vi "Dashboard_Main_Fixed_1280_768.vi"() -> ()   [LabVIEW 2023]
uses:
  2025ReefBot/Intake/IntakeStates.ctl
  2025ReefBot/NewAuto/NewAutoStepTypeEnum.ctl
  <vilib>/event_ctls.llb/eventvkey.ctl
  Dash_Globals.vi
  <vilib>/Rock Robotics/Network Tables/NT Read Boolean.vi
  <vilib>/Rock Robotics/Network Tables/NT Write Boolean.vi
  <vilib>/Rock Robotics/WPI/Dashboard/WPI_DashboardLogging Global.vi
  <vilib>/Rock Robotics/WPI/ThirdParty/JAS_Junk/TrajLib/Trajectory_Library.lvlib
panel:
  in  "Camera Settings Right":T1={"Frame Rate"=30, "Compression"=30, "Size"=1, "DB Camera Config"=FALSE} {"Frame Rate" scale=1.0..30.0; "Compression" scale=100.0..-1.0; "Size" items=["640x480", "320x240", "160x120"]}
  in  "Camera Name Right":string(combo)="No Camera Selection"
  out "Camera Perf":string
  in  "Camera Settings":T1={"Frame Rate"=30, "Compression"=30, "Size"=1, "DB Camera Config"=FALSE} {"Frame Rate" scale=1.0..30.0; "Compression" scale=100.0..-1.0; "Size" items=["640x480", "320x240", "160x120"]}
  in  "TCP":refnum<k5>
  in  "Rec Mode":enum32{"Stop", "Record", "Playback"}(radio)
  out "Robot IP":string
  out "Image Message":string="Timeout in Camera Communications"
  in  "Dashboard Tab":T2(tab)
  out "Human Fast Turn":bool
  out "H Traj Orient Deg":dbl format="%11.2f"
  out "H Traj Y Ft":dbl format="%11.2f"
  out "H Traj X Ft":dbl format="%11.2f"
  out "Human Slow Mode":bool
  out "Human Field Orient":bool
  out "A String":string
  out "P3":dbl format="%11.2f"
  out "Function":T3
  out "A Step":i64 format="%11.0f"
  out "P2":dbl format="%11.2f"
  out "P1":dbl format="%11.2f"
  out "TO":dbl format="%11.2f"
  out "Vision Targets Found":bool
  out "Climb Position":dbl format="%15.2f"
  out "Climb Status":string
  out "Fully Pulled":bool
  out "Fully Reached":bool
  out "Intake State":T4
  out "Have Algae":bool
  out "Have Coral":bool
  out "W PV":dbl(slide) scale=-90.0..90.0
  out "W SP":dbl(slide) scale=-90.0..90.0
  out "W Hi Clamp":bool
  out "W Lo Clamp":bool
  out "W On Tgt":bool
  out "W Motor":dbl format="%11.2f"
  out "W Pos Deg":dbl format="%12.1f"
  out "W Dmd Deg":dbl format="%12.1f"
  out "I PV":dbl(slide) scale=0.0..26.0
  out "I SP":dbl(slide) scale=0.0..26.0
  out "I Lo Clamp":bool
  out "I Lo Lim":bool
  out "I Hi Lim":bool
  out "I On Tgt":bool
  out "I Motor":dbl format="%11.2f"
  out "I Pos In":dbl format="%12.1f"
  out "I Dmd In":dbl format="%12.1f"
  in  "Select Auto":string(combo)="Select Autonomous ..."
  out "NT Connection":bool
  out "Mode":T5(ring)=enum."Auto Disabled"
  out "Right Camera Perf":cluster{"Bandwidth (Mbps)":dbl, "FPS":dbl}
  out "Selected Auto":string
  out "O PV":dbl(slide) scale=0.0..52.0
  out "O SP":dbl(slide) scale=0.0..52.0
  out "O Lo Lim":bool
  out "O Hi Lim":bool
  out "O On Tgt":bool
  out "O Motor":dbl format="%11.2f"
  out "O Pos In":dbl format="%12.1f"
  out "O Dmd In":dbl format="%12.1f"
  out "Camera Image Right":T6(plugin-control)
  out "AlgaeIntakeFB":dbl
  out "AlgaeHoldFB":dbl
  in  "AlgaeIntake":dbl
  in  "AlgaeHold":dbl
  in  "AlgaeTune":bool
  out "Max Amb FB":dbl
  in  "Max Amb":dbl
  out "I Orient Deg FB":dbl
  in  "Init Orient Deg":dbl
  out "InitYPosFt FB":dbl
  in  "InitYPos Ft":dbl
  in  "Vision Update":bool
  out "InitXPos Ft FB":dbl
  in  "InitXPos Ft":dbl
  out "RL Enable FB":bool
  in  "RL Enable":bool
  out "Y Acc M/S2 FB":dbl
  in  "Y Acc M/S2":dbl
  in  "RL Update":bool
  out "X Acc M/S2 FB":dbl
  in  "X Acc M/S2":dbl
  in  "RA Update":bool
  out "R Starting Angle FB":dbl
  in  "R Starting Angle":dbl
  in  "LQR":bool
  in  "Filter":bool
  out "Wrist Chart":T7(graph)
  out "Kp Calc":dbl
  out "Kg FB":dbl
  in  "Kg":dbl
  out "Kd FB":dbl format="%#_7g"
  in  "Kd":dbl format="%#_7g"
  out "Output Max FB":dbl
  in  "Output Max":dbl
  out "Output DB FB":dbl
  in  "Output DB":dbl
  out "Error DB FB":dbl
  in  "Error DB":dbl
  in  "WR Tune Update":bool
  out "Error Thres FB":dbl
  in  "Error Thres":dbl
  out "Filt FB":bool
  out "LQR FB":bool
  in  "Test Slider":dbl(slide) scale=0.0..100.0 scale format="%#_3g"
  in  "On/Off":bool caption="Solenoid"
  in  "Test Name":u16(ring) items=["Select the test to run..."]
  in  "Test Tree":string(tree)
  in  "Motor":cluster{"Value":dbl, "Enable":bool} {"Value" scale=-1.0..1.0 scale format="%#_3g"}
  out "Progress":T8 {"Test Progress" scale=0.0..100.0}
  in  "Rev/Fwd":cluster{"Forward":bool, "Reverse":bool}
  in  "Test Ring":u16(ring) items=["Monochrome", "Color"]
  in  "CheckList":i32(listbox)
  out "Tree":string(tree)
  out "Camera Image":T6(plugin-control)
  out "Background":bool
  in  "Camera Name":string(combo)="No Camera Selection"
  # "HW"
  # "HW"
  # "Human"
  # "Auto"
  # "VISION"
  # "CLIMB"
  # "INTAKE"
  # "WRIST"
  # "INNER ELEV"
  # "OUTER ELEV"
  # "Vision Tuning"
  # "Drive Rate Limiting"
  # "Initial Robot Angle"
  # "Wrist Tuning"
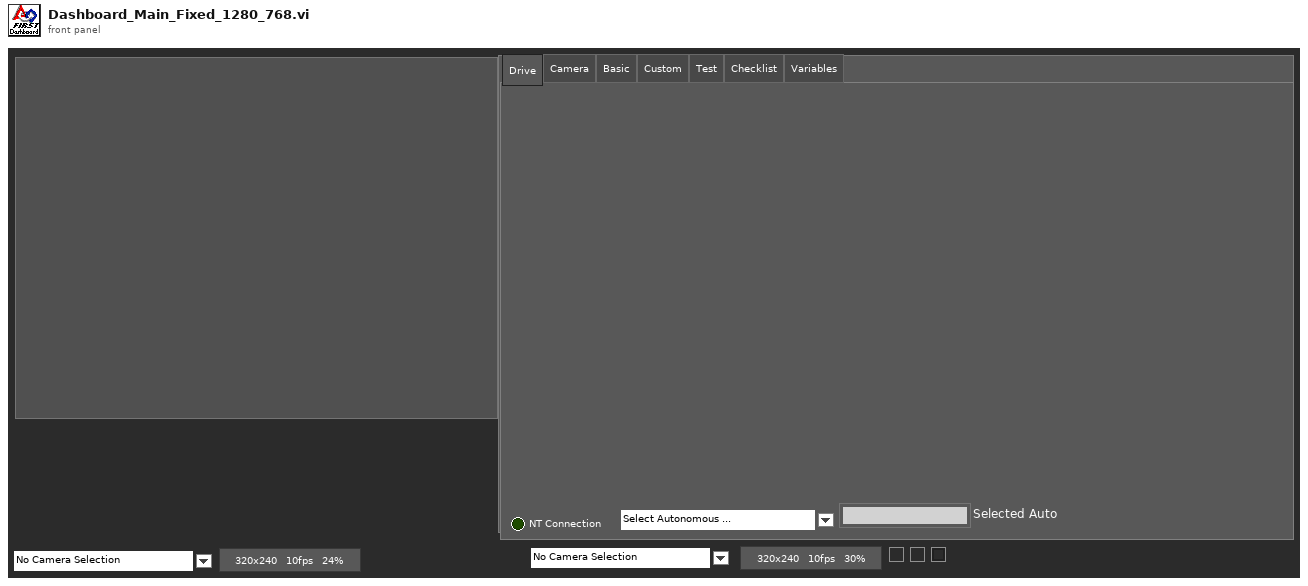
[diagram p1: front panel]
types:
  T1 = cluster{"Frame Rate":i32, "Compression":i32, "Size":u16, "DB Camera Config":bool}
  T2 = enum32{"Drive", "Camera", "Basic", "Custom", "Test", "Checklist", "Variables"}
  T3 = typedef "NewAutoStepTypeEnum.ctl" = enum16{"DriveStraight", "DriveTurn", "FollowAbsoluteTrajectory", "FollowRelativeTrajectory", "AutoWait", "ElevToRest", "ElevToFloor", "ElevToSource", "ElevToL1", "ElevToL2", "ElevToL3", "ElevToL4", "ElevToAlgae1", "ElevToAlgae2", "ElevToBarge", "ElevCancel", "IntakeCoral", "IntakeAlgae", "IntakeDepositCoral", "IntakeDepositAlgae", "IntakeCancel", "ElevRestWait", "ElevFloorWait", "ElevSourceWait", "ElevL1Wait", "ElevL2Wait", "ElevAlgae1Wait", "ElevL3Wait", "ElevAlgae2Wait", "ElevL4Wait", "ElevBargeWait", "IntakeWait", "FollowAbsTrajWithTimedCmd", "FollowRelTrajWithTimedCmd"}
  T4 = typedef "IntakeStates.ctl" = enum16{"Start", "WaitForCommand", "IntakeCoral", "IntakeAlgae", "WaitForCoral", "WaitForAlgae", "DepositCoral", "DepositAlgae", "DepositCoralTimer", "DepositAlgaeTimer"}
  T5 = enum8{"Tele-Op Disabled", "Tele-Op Enabled", "Auto Disabled", "Auto Enabled", "Test Disabled", "Test Enabled", "Disconnected", "No Code", "E-Stop"}
  T6 = typedef "IMAQ Image.ctl" = refnum<image>
  T7 = cluster{"WristSetpointDeg":dbl, "WristPosDeg":dbl, "WristMotorDmd":dbl, "WristGravityCompMotorDmd":dbl}
  T8 = cluster{"Test Progress":u8, "Test Progress Text":string}
  T9 = cluster{"Save Path":path, "Interval (s)":dbl, "Keep":i32}
  T10 = typedef "Image Type" = u32
  T11 = enum32{"Drive", "Camera", "Basic", "Custom", "Test", "Commands", "Checklist", "Variables"}
  T12 = cluster{"Error Strings":string, "Disable Counts":cluster{u16, u16}, "Rail Faults":cluster{u16, u16, u16}, "Robot IP":string, "DB Mode":u8, "Event Info":cluster{"Name":string, "Type":u8, "Number":u16, "Replay":u8}}
  T13 = cluster{"Storage":cluster{"Disk Free":u64, "RAM Block":u32, "RAM free":u32}, "CPU Utilization":cluster{"CPU % ISR":sgl, "CPU % Time Crit":sgl, "CPU % Timed Str":sgl, "CPU % High":sgl, "CPU % Above":sgl, "CPU % Normal":sgl, "CPU % Low":sgl}, "CAN":cluster{"% Bus Utilization":sgl, "Bus Off Cnt":u32, "TX_FIFO Full Cnt":u32, "Receive Error Cnt":u8, "Transmit Error Cnt":u8}, "HID":cluster{"HID Outputs":u32, "Rumble Low":u16, "Rumble High":u16}[]}
  T14 = cluster{"Status bits":cluster{"Test Mode":bool, "Autonomous":bool, "Enabled":bool, "Code Start":bool, "Brownout":bool, "Reserved 2":bool, "Reserved 3":bool, "E-Stop":bool}, "Code Trace":cluster{"Disabled":bool, "TeleOp":bool, "Auto":bool, "Test":bool}, "Controller Type":enum16{"unknown", "cRIO", "roboRio"}, "Code?":enum16{"unknown", "noCode", "code"}, "Battery V":dbl}
  T15 = cluster{"Control Bits":cluster{"TestMode":bool, "Autonomous":bool, "Enabled":bool, "FMS Present":bool, bool, bool, bool, "E-Stop":bool}, "Team Station ":u8, "Countdown":sgl, "Joystick Values":cluster{"Axes":dbl[], "Buttons":bool[], "POVs":i16[]}[]}
  T16 = cluster{"Camera Image":refnum<vi>, "Dashboard Tab":refnum<vi>, "Background":refnum<vi>, "Rec Mode":refnum<vi>, "Test Slider":refnum<vi>, "On/Off ":refnum<vi>, "Test Ring":refnum<vi>, "Rev/Fwd":refnum<vi>, "Test Name":refnum<vi>, "Motor":refnum<vi>, "Progress":refnum<vi>, "CheckList":refnum<vi>, "Tree":refnum<vi>, "Test Tree":refnum<vi>, "Camera Settings":refnum<vi>, "Camera Name":refnum<vi>, "Camera Perf":refnum<vi>, "Camera Settings Right":refnum<vi>, "Camera Name Right":refnum<vi>, "Camera Image Right":refnum<vi>}
  T17 = cluster{"Global Rectangle":i32[], "Contours":cluster{"Contour Type":u32, "ROI Type":u32, "Points":i32[]}[]}
  T18 = cluster{"Camera Name":string, string, "Saved DB Images Info":cluster{"Save Path":path, "Interval (s)":dbl, "Keep":i32}}
  T19 = cluster{"Camera Name Right":string, string, "Saved DB Images Info":cluster{"Save Path":path, "Interval (s)":dbl, "Keep":i32}}
  T20 = cluster{"Operation":enum16{"Update", "Clear"}, "Color Box":u32}[]
  T21 = typedef "eventvkey.ctl" = enum16{"ASCII", "Enter", "Return", "Shift", "Ctrl", "Alt", "Cmd", "Opt", "Caps", "NumLock", "Clear", "Break", "Up", "Down", "Left", "Right", "Insert", "Delete", "Home", "End", "PageUp", "PageDown", "Escape", "Help", "Pause", "ScrollLock", "F1", "F2", "F3", "F4", "F5", "F6", "F7", "F8", "F9", "F10", "F11", "F12", "F13", "F14", "F15", "F16", "F17", "F18", "F19", "F20", "F21", "F22", "F23", "F24", "Play", "VolumeUp", "VolumeDown", "Mute", "Two Byte Char"}
  T22 = cluster{"Image Size":bool, "Image Type":bool, "Pixel Value":bool, "ROI Information":bool, "Zoom Factor":bool}
  T23 = cluster{"Operation":enum16{"Update", "Clear"}, "Color Box":u32}
  T24 = cluster{"Shift":bool, "Ctrl":bool, "Alt":bool, "Cmd":bool, "Opt":bool}
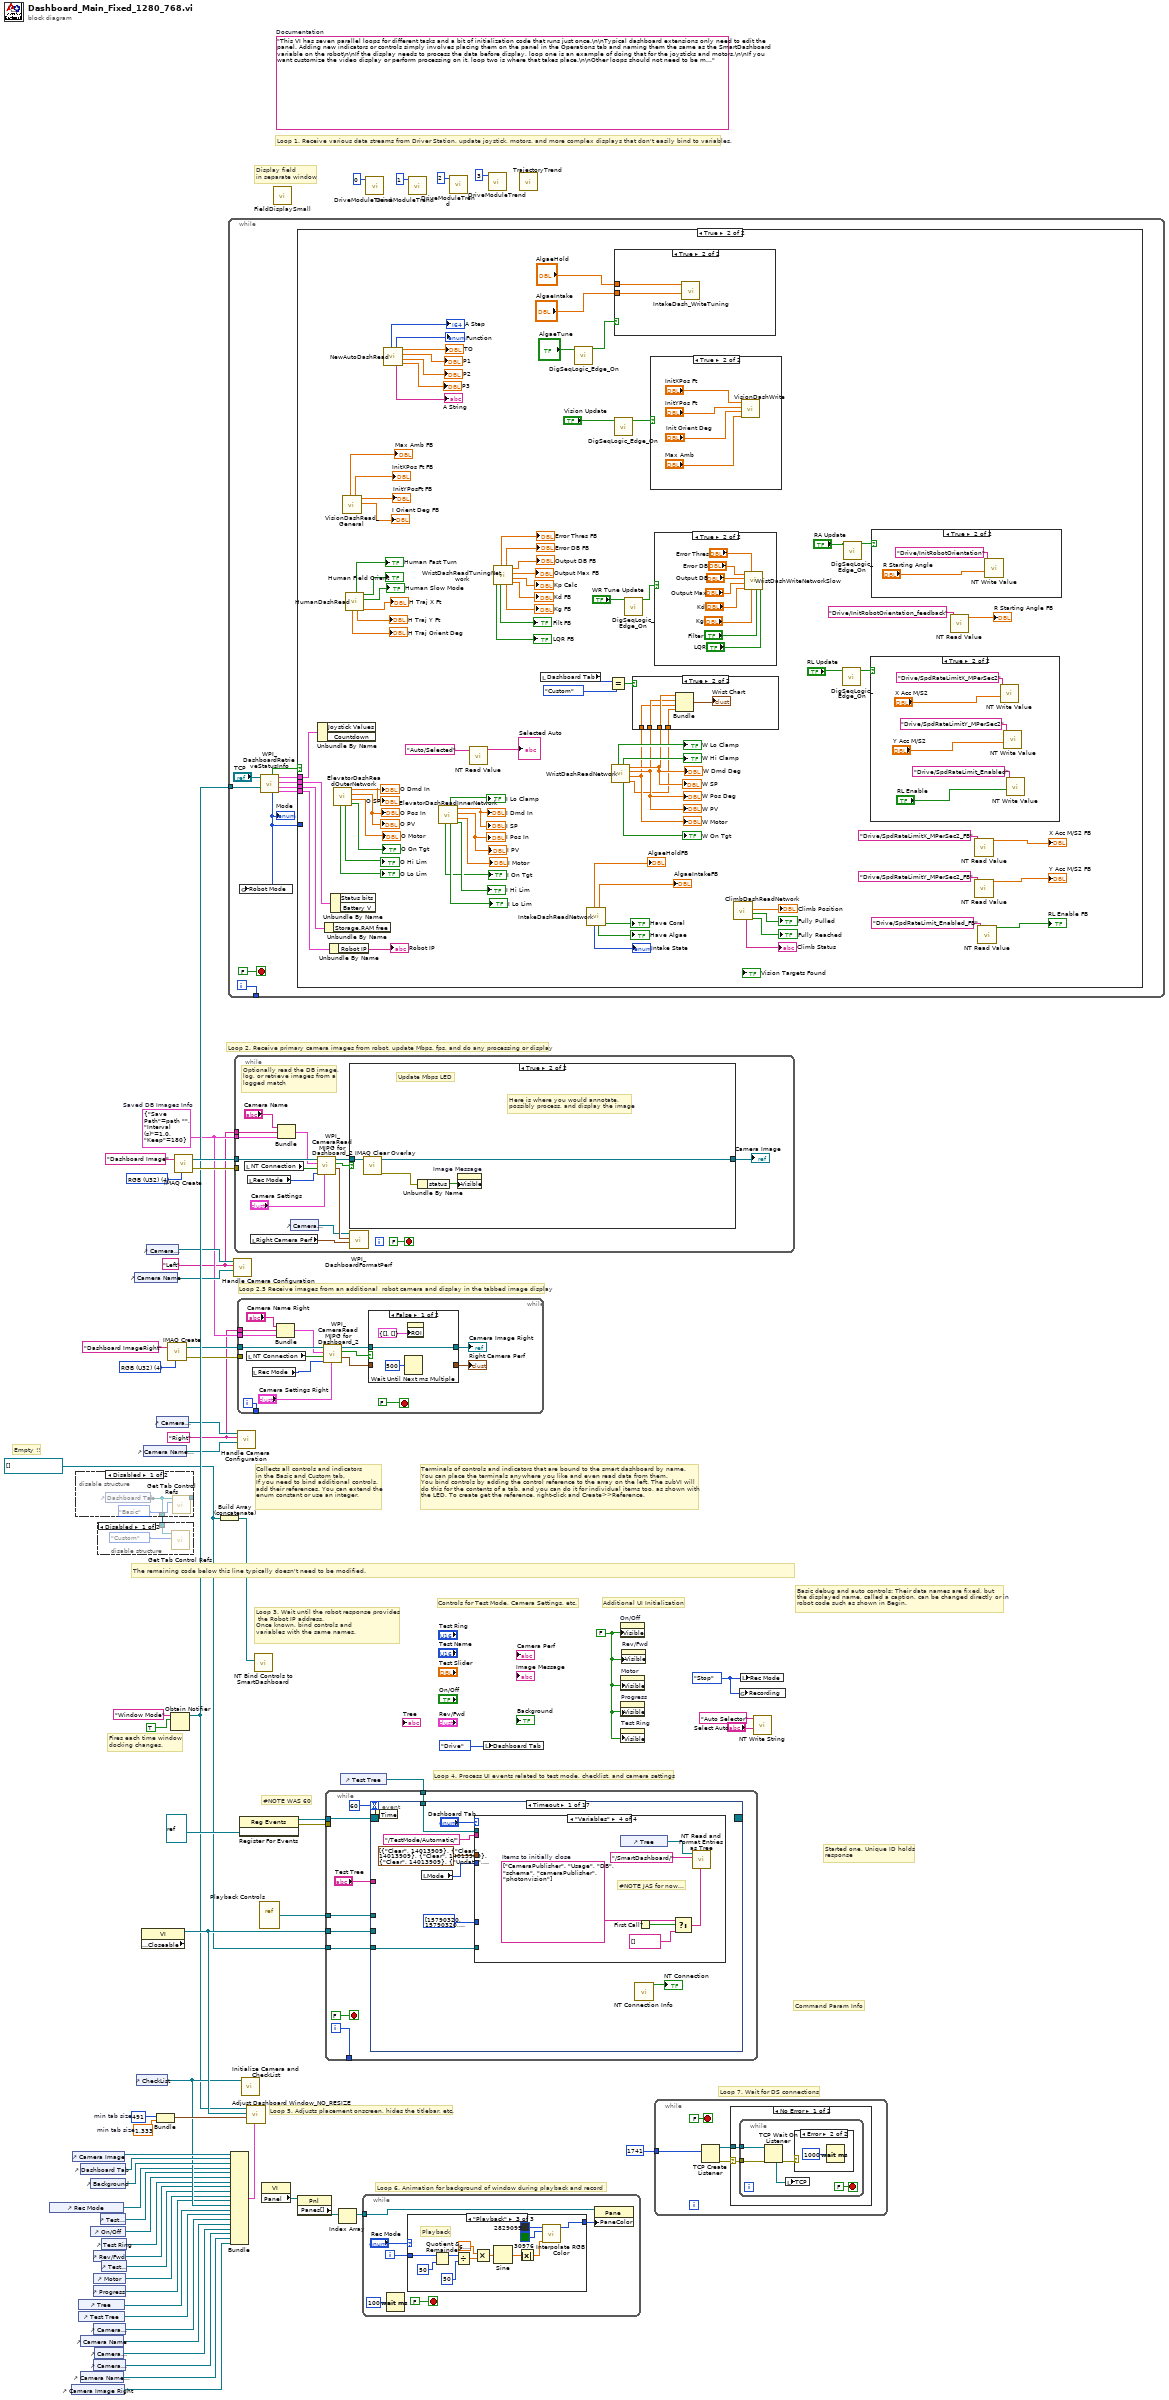
[diagram p0: block diagram]
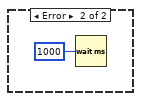
[diagram p6: hidden frame]
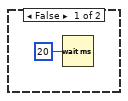
[diagram p7: hidden frame]
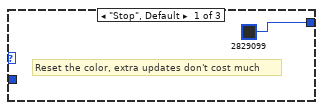
[diagram p14: hidden frame]
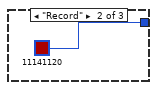
[diagram p15: hidden frame]
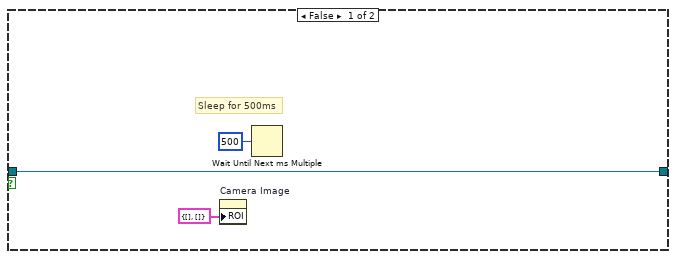
[diagram p16: hidden frame]
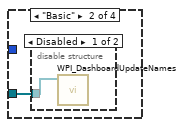
[diagram p18: hidden frame]
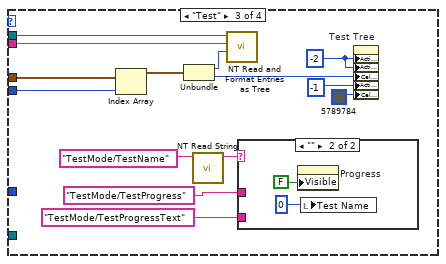
[diagram p20: hidden frame]
diagram:
  w5 = refnum<vi>[] [] ("ControlsOnPage")
  w8 = T9 {"Save Path"=path "", "Interval (s)"=1.0, "Keep"=180}  # Saved DB Images Info
  w7 = "Right"
  w6 = "Left"
  w16 = T10 4 items=["Grayscale (U8)", "Grayscale (I16)", "Grayscale (SGL)", "Complex (CSG)", "RGB (U32)", "HSL (U32)", "RGB (U64)"] ("Image Type")
  w44 = 491  # min tab size
  w43 = 1.333  # min tab size
  w50 = enum32{"Stop", "Record", "Playback"}."Stop" ("Rec Mode")
  w28 = FALSE ("Visible")
  (unwired) "This VI has seven parallel loops for different tasks and a bit of initialization code that runs just once.\n\nTypical dashboard extensions only need to edit the panel. Adding new indicators or controls simply involves placing them on the panel in the Operations tab and naming them the same as the SmartDashboard variable on the robot\n\nIf the display needs to process the data before display, loop one is an example of doing that for the joysticks and motors.\n\nIf you want customize the video display or perform processing on it, loop two is where that takes place.\n\nOther loops should not need to be modified. They are pretty standard, and document the task they perform."  # Documentation
  w64 = T10 4 items=["Grayscale (U8)", "Grayscale (I16)", "Grayscale (SGL)", "Complex (CSG)", "RGB (U32)", "HSL (U32)", "RGB (U64)"] ("Image Type")
  # "#NOTE WAS 60"
  # "Empty !!"
  # "Display field\nin separate window"
  # "Loop 2.5 Receive images from an additional  robot camera and display in the tabbed image display"
  # "Command Param Info"
  # "Started one, Unique ID holds\nresponse"
  # "Loop 7. Wait for DS connections"
  # "Basic debug and auto controls: Their data names are fixed, but\nthe displayed name, called a caption, can be changed directly or in\nrobot code such as shown in Begin."
  # "Controls for Test Mode, Camera Settings, etc."
  # "Additional UI Initialization"
  # "Loop 6. Animation for background of window during playback and record"
  # "Fires each time window\ndocking changes."
  # "Collects all controls and indicators\nin the Basic and Custom tab.\nIf you need to bind additional controls,\nadd their references. You can extend the\nenum constant or use an integer."
  # "The remaining code below this line typically doesn't need to be modified."
  # "Loop 4. Process UI events related to test mode, checklist, and camera settings"
  # "Terminals of controls and indicators that are bound to the smart dashboard by name.\nYou can place the terminals anywhere you like and even read data from them.\nYou bind controls by adding the control reference to the array on the left. The subVI will\ndo this for the contents of a tab, and you can do it for individual items too, as shown with\nthe LED. To create get the reference, right-click and Create>>Reference."
  # "Loop 3. Wait until the robot response provides\n the Robot IP address.\nOnce known, bind controls and\nvariables with the same names."
  # "Loop 5. Adjusts placement onscreen, hides the titlebar, etc."
  # "Loop 1. Receive various data streams from Driver Station, update joystick, motors, and more complex displays that don't easily bind to variables."
  # "Loop 2. Receive primary camera images from robot, update Mbps, fps, and do any processing or display"
  n1 = control-ref of="Rec Mode"() -> (w34:refnum<vi>)
  n2 = control-ref of="Camera Image Right"() -> (w9:refnum<vi>)
  n3 = control-ref of="Camera Image"() -> (w46:refnum<vi>)
  n4 = disable-structure shown="Disabled" {
    disable-tunnel: [w67 _] -> w48
    disable-tunnel: [w66 _] -> _
    frame Disabled {
      n5 = control-ref of="Dashboard Tab"() -> (w67:refnum<vi>)
      n6 = call <vilib>:"Get Tab Control Refs.vi"("Page Index"=T11."Basic" ("Dashboard Tab"), "TabControl in"=w67) -> ("ControlsOnPage"=w66:refnum<vi>[])  [unwired: 9 in]
    }
    frame Enabled {
    }
  }
  n7 = control-ref of="Tree"() -> (w38:refnum<vi>)
  n8 = control-ref of="Test Tree"() -> (w37:refnum<vi>)
  n9 = control-ref of="Dashboard Tab"() -> (w45:refnum<vi>)
  n10 = control-ref of="Camera Name"() -> (w21:refnum<vi>)
  n11 = control-ref of="Camera Name Right"() -> (w10:refnum<vi>)
  n12 = control-ref of="Background"() -> (w41:refnum<vi>)
  n13 = control-ref of="On/Off"() -> (w32:refnum<vi>)
  n14 = control-ref of="Progress"() -> (w29:refnum<vi>)
  n15 = control-ref of="Camera Settings"() -> (w22:refnum<vi>)
  n16 = control-ref of="Camera Settings Right"() -> (w11:refnum<vi>)
  n17 = control-ref of="Rev/Fwd"() -> (w30:refnum<vi>)
  n18 = control-ref of="Motor"() -> (w35:refnum<vi>)
  n19 = control-ref of="Camera Perf"() -> (w20:refnum<vi>)
  n20 = disable-structure shown="Disabled" {
    disable-tunnel: w48 -> [w69 _]
    frame Disabled {
      n21 = call <vilib>:"Get Tab Control Refs.vi"("Page Index"=T11."Custom" ("Dashboard Tab"), "TabControl in"=w69) -> ()  [unwired: 9 in, 1 out]
    }
    frame Enabled {
    }
  }
  n22 = control-ref of="Test Slider"() -> (w33:refnum<vi>)
  n23 = control-ref of="Test Ring"() -> (w31:refnum<vi>)
  n24 = control-ref of="Test Name"() -> (w36:refnum<vi>)
  n25 = control-ref of="Camera Name"() -> (w23:refnum<vi>)
  n26 = control-ref of="CheckList"() -> (w39:refnum<vi>)
  n27 = property class="VI" props=["Front Panel.Closeable"]() -> (reference out=w49:refnum<vi>)  [unwired: 2 in, 2 out]
  n28 = control-ref of="Camera Name Right"() -> (w12:refnum<vi>)
  n29 = control-ref of="Camera Settings"() -> (w24:refnum<vi>)
  n30 = control-ref of="Camera Settings Right"() -> (w13:refnum<vi>)
  n31 = Bundle("min tab size"=w44, "min tab size"=w43) -> (w42:cluster{"min tab size":i32, "min tab size":dbl})  [unwired: 1 in]
  n32 = call "IMAQ Create"("Image Name"="Dashboard ImageRight", "Image Type"=w16) -> ("New Image"=w15:T6, "error out"=w14:errorcluster)  [unwired: 2 in, 1 out]
  n33 = Obtain Notifier(name (unnamed)="Window Mode", notification data type=TRUE) -> (notifier out=w27:refnum<notifier>)  [unwired: 2 in, 2 out]
  n34 = call "IMAQ Create"("Image Name"="Dashboard Image", "Image Type"=w64) -> ("New Image"=w62:T6, "error out"=w61:errorcluster)  [unwired: 2 in, 1 out]
  n35 = Build Array (concatenate)(w5) -> (w47:refnum<vi>[])
  n36 = while {
    tunnel: [w78] -> _
    tunnel: w27 -> [w71]
    i -> [w78]
    stop <- FALSE stop-if-true
    n37 = call <vilib>:"WPI_DashboardRetrieveStatusInfo.vi"("Window Mode Notifier"=w71, "TCP Cnx"="TCP") -> ("Power and Errors"=w73:T12, "Robot Metrics"=w76:T13, "Status Info"=w77:T14, "Control Info"=w74:T15, "Robot Mode"=w70:T5, "Process?"=w75:bool)  [unwired: 4 in]
    "Mode" <- w70
    n38 = global write "Dash_Globals.vi" "Robot Mode"(w70) -> ()
    n39 = case shown="True" w75 {
      tunnel: w77 -> [_ w165]
      tunnel: w76 -> [_ w164]
      tunnel: w74 -> [_ w163]
      tunnel: w73 -> [_ w162]
      tunnel: w70 -> [_ _]
      frame False {
        n40 = Wait (ms)(milliseconds to wait=u32 20) -> ()  [unwired: 1 out]
      }
      frame True {
        n41 = Unbundle By Name(w163) -> ()  [unwired: 2 out]
        n42 = Unbundle By Name(w164) -> ()  [unwired: 1 out]
        n43 = Unbundle By Name(w162) -> ("Robot IP"=→"Robot IP":string)
        n44 = Unbundle By Name(w165) -> ()  [unwired: 2 out]
        n45 = call "ElevatorDashReadOuterNetwork.vi"() -> ("OuterOnTarget"=→"O On Tgt":bool, "OuterMotorOutput"=→"O Motor":dbl, "OuterPositionHeight"=→"O PV" →"O Pos In":dbl, "OuterPosDemandHeight"=→"O SP" →"O Dmd In":dbl, "OuterHighLimitSwitch"=→"O Hi Lim":bool, "OuterLowLimitSwitch"=→"O Lo Lim":bool)  [unwired: 6 in]
        n46 = call "VisionDashRead_General.vi"() -> ("InitOrientDeg"=→"I Orient Deg FB":dbl, "InitYFt"=→"InitYPosFt FB":dbl, "InitXFt"=→"InitXPos Ft FB":dbl, "MaxAmbiguity"=→"Max Amb FB":dbl)  [unwired: 4 in, 4 out]
        n47 = call "HumanDashRead.vi"() -> ("TrajDestX_Ft"=→"H Traj X Ft":dbl, "SlowMode"=→"Human Slow Mode":bool, "FieldOriented"=→"Human Field Orient":bool, "TrajDestY_Ft"=→"H Traj Y Ft":dbl, "FastMode"=→"Human Fast Turn":bool, "TrajDestAng_Deg"=→"H Traj Orient Deg":dbl)  [unwired: 5 in, 1 out]
        n48 = call "NewAutoDashRead.vi"() -> ("P3"=→"P3":dbl, "P2"=→"P2":dbl, "P1"=→"P1":dbl, "Timeout"=→"TO":dbl, "StepString"=→"A String":string, "StepType"=→"Function":T3, "StepIndex"=→"A Step":i64)  [unwired: 5 in]
        n49 = call "ElevatorDashReadInnerNetwork.vi"() -> ("Stage3HighLimitSwitch"=→"I Hi Lim":bool, "Stage3MotorOutput"=→"I Motor":dbl, "Stage3PositionHeight"=→"I Pos In" →"I PV":dbl, "Stage3PosDemandHeight"=→"I Dmd In" →"I SP":dbl, "Stage3LowLimitSwitch"=→"I Lo Lim":bool, "Stage3LowWristClampActive"=→"I Lo Clamp":bool, "Stage3OnTarget"=→"I On Tgt":bool)  [unwired: 5 in]
        n50 = call-poly <vilib>:"NT Read Value.vi"("name"="Auto/Selected") -> ("value"=→"Selected Auto":string)  [unwired: 8 in, 2 out]
        n51 = call "WristDashReadTuningNetwork.vi"() -> ("Tune_Kd"=→"Kd FB":dbl, "Tune_Kp"=→"Kp Calc":dbl, "Tune_OutMax"=→"Output Max FB":dbl, "Tune_OutDb"=→"Output DB FB":dbl, "Tune_Kg"=→"Kg FB":dbl, "Tune_ErrDb"=→"Error DB FB":dbl, "FilterDerivative"=→"Filt FB":bool, "Tune_ErrThres"=→"Error Thres FB":dbl, "UseLQR"=→"LQR FB":bool)  [unwired: 3 in]
        n52 = local read "Dashboard Tab"() -> (w113:T2)
        n53 = call <vilib>:"DigSeqLogic_Edge_On.vi"("Input"="AlgaeTune") -> ("On Edge"=w85:bool)  [unwired: 10 in]
        n54 = call "IntakeDashReadNetwork.vi"() -> ("HaveCoralSensor"=→"Have Coral":bool, "HaveAlgaeSensor"=→"Have Algae":bool, "AlgaeIntake"=→"AlgaeIntakeFB":dbl, "CurrentState"=→"Intake State":T4, "AlgaeHold"=→"AlgaeHoldFB":dbl)  [unwired: 4 in, 3 out]
        n55 = Equal?(x=w113, y=T2."Custom") -> (x = y?=w114:bool)
        n56 = call "WristDashReadNetwork.vi"() -> ("WristGravityCompMotorDmd"=w106:dbl, "WristMotorDmd"=w109:dbl, "WristPosDeg"=w110:dbl, "WristSetpointDeg"=w111:dbl, "WristAtSetpoint"=→"W On Tgt":bool, "WristProtectHighClampActive"=→"W Hi Clamp":bool, "WristProtectLowClampActive"=→"W Lo Clamp":bool)  [unwired: 5 in]
        "W Dmd Deg" <- w111
        "W Pos Deg" <- w110
        "W Motor" <- w109
        "W SP" <- w111
        "W PV" <- w110
        n57 = case shown="True" w85 {
          tunnel: "AlgaeHold" -> [_ w167]
          tunnel: "AlgaeIntake" -> [_ w166]
          frame False {
          }
          frame True {
            n58 = call "IntakeDash_WriteTuning.vi"("AlgaeIntake"=w166, "Hold"=w167) -> ()  [unwired: 10 in]
          }
        }
        n59 = call <vilib>:"DigSeqLogic_Edge_On.vi"("Input"="Vision Update") -> ("On Edge"=w104:bool)  [unwired: 10 in]
        n60 = call <vilib>:"DigSeqLogic_Edge_On.vi"("Input"="WR Tune Update") -> ("On Edge"=w116:bool)  [unwired: 10 in]
        n61 = case shown="True" w114 {
          tunnel: w111 -> [_ w175]
          tunnel: w110 -> [_ w174]
          tunnel: w109 -> [_ w173]
          tunnel: w106 -> [_ w172]
          frame False {
          }
          frame True {
            n62 = Bundle("WristSetpointDeg"=w175, "WristPosDeg"=w174, "WristMotorDmd"=w173, "WristGravityCompMotorDmd"=w172) -> (→"Wrist Chart":T7)  [unwired: 1 in]
          }
        }
        n63 = case shown="True" w104 {
          frame False {
          }
          frame True {
            n64 = call "VisionDashWrite.vi"("MaxAmbiguity"="Max Amb", "InitialOrientationDeg"="Init Orient Deg", "InitialYPositionFt"="InitYPos Ft", "InitialXPositionFt"="InitXPos Ft") -> ()  [unwired: 8 in]
          }
        }
        n65 = case shown="True" w116 {
          frame False {
          }
          frame True {
            n66 = call "WristDashWriteNetworkSlow.vi"("UseLQR"="LQR", "FilterDerivative"="Filter", "Tune_Kg"="Kg", "Tune_ErrThres"="Error Thres", "Tune_Kd"="Kd", "Tune_OutMax"="Output Max", "Tune_OutDb"="Output DB", "Tune_ErrDb"="Error DB") -> ()  [unwired: 4 in]
          }
        }
        n67 = call "ClimbDashReadNetwork.vi"() -> ("ReachLimit"=→"Fully Reached":bool, "PullLimit"=→"Fully Pulled":bool, "SensorPosition"=→"Climb Position":dbl, "ClimbStatus"=→"Climb Status":string)  [unwired: 7 in, 1 out]
        n68 = call <vilib>:"DigSeqLogic_Edge_On.vi"("Input"="RL Update") -> ("On Edge"=w130:bool)  [unwired: 10 in]
        n69 = call <vilib>:"DigSeqLogic_Edge_On.vi"("Input"="RA Update") -> ("On Edge"=w132:bool)  [unwired: 10 in]
        n70 = case shown="True" w130 {
          frame False {
          }
          frame True {
            n71 = call-poly <vilib>:"NT Write Value.vi"("value"="X Acc M/S2", "name"="Drive/SpdRateLimitX_MPerSec2") -> ()  [unwired: 9 in, 1 out]
            n72 = call-poly <vilib>:"NT Write Value.vi"("value"="Y Acc M/S2", "name"="Drive/SpdRateLimitY_MPerSec2") -> ()  [unwired: 9 in, 1 out]
            n73 = call-poly <vilib>:"NT Write Value.vi"("value"="RL Enable", "name"="Drive/SpdRateLimit_Enabled") -> ()  [unwired: 9 in, 1 out]
          }
        }
        n74 = case shown="True" w132 {
          frame False {
          }
          frame True {
            n75 = call-poly <vilib>:"NT Write Value.vi"("value"="R Starting Angle", "name"="Drive/InitRobotOrientation") -> ()  [unwired: 9 in, 1 out]
          }
        }
        n76 = call-poly <vilib>:"NT Read Value.vi"("name"="Drive/InitRobotOrientation_feedback") -> ("value"=→"R Starting Angle FB":dbl)  [unwired: 8 in, 2 out]
        n77 = call-poly <vilib>:"NT Read Value.vi"("name"="Drive/SpdRateLimitX_MPerSec2_FB") -> ("value"=→"X Acc M/S2 FB":dbl)  [unwired: 8 in, 2 out]
        n78 = call-poly <vilib>:"NT Read Value.vi"("name"="Drive/SpdRateLimitY_MPerSec2_FB") -> ("value"=→"Y Acc M/S2 FB":dbl)  [unwired: 8 in, 2 out]
        n79 = call-poly <vilib>:"NT Read Value.vi"("name"="Drive/SpdRateLimit_Enabled_FB") -> ("value"=→"RL Enable FB":bool)  [unwired: 8 in, 2 out]
      }
    }
  }
  n80 = Bundle("Camera Image"=w46, "Dashboard Tab"=w45, "Background"=w41, "Rec Mode"=w34, "Test Slider"=w33, "On/Off"=w32, "Test Ring"=w31, "Rev/Fwd"=w30, "Test Name"=w36, "Motor"=w35, "Progress"=w29, "CheckList"=w39, "Tree"=w38, "Test Tree"=w37, "Camera Settings"=w22, "Camera Name"=w21, "Camera Perf"=w20, "Camera Settings Right"=w11, "Camera Name Right"=w10, "Camera Image Right"=w9) -> (w40:T16)  [unwired: 1 in]
  n81 = call "Handle Camera Configuration.vi"("CameraNameRef"=w23, "Display Name"=w6, "ClusterRef"=w24) -> ()  [unwired: 9 in]
  n82 = while {
    tunnel: w62 -> [w206]
    tunnel: w61 -> [_]
    tunnel: w8 -> [w199]
    tunnel: w6 -> [w196]
    stop <- FALSE stop-if-true
    # "Optionally read the DB image,\nlog, or retrieve images from a\nlogged match"
    n83 = local read "NT Connection"() -> (w200:bool)
    n84 = local read "Rec Mode"() -> (w203:enum32{"Stop", "Record", "Playback"})
    n85 = local read "Right Camera Perf"() -> (w194:cluster{"Bandwidth (Mbps)":dbl, "FPS":dbl})
    n86 = Bundle("Camera Name"="Camera Name", w196, "Saved DB Images Info"=w199) -> (w198:T18)  [unwired: 1 in]
    n87 = control-ref of="Camera Perf"() -> (w193:refnum<vi>)
    n88 = call <vilib>:"WPI_CameraRead MJPG for Dashboard_2.vi"("Camera Settings"="Camera Settings", "Rec Mode"=w203, "NT Connection"=w200, "Capture Info"=w198, "Image in"=w206) -> ("perf info"=w195:cluster{"Bandwidth (Mbps)":dbl, "fps":dbl}, "Active"=w204:bool, "Image\\ out"=w205:T6)  [unwired: 4 in]
    n89 = case shown="True" w204 {
      tunnel: w205 -> [w209 w212]
      tunnel: [w209 w211] -> w201
      frame False {
        # "Sleep for 500ms"
        n90 = property on="Camera Image" class="ImageControl"("ROI"=T17 {"Global Rectangle"=[], "Contours"=[]}) -> ()  [unwired: 2 in, 2 out]
        n91 = Wait Until Next ms Multiple(millisecond multiple=u32 500) -> ()  [unwired: 1 out]
      }
      frame True {
        # "Here is where you would annotate,\npossibly process, and display the image"
        # "Update Mbps LED"
        n92 = call "IMAQ Clear Overlay"("Image"=w212) -> ("error out"=w213:errorcluster, "Image Out"=w211:T6)  [unwired: 2 in, 7 out]
        n93 = Unbundle By Name(w213) -> ("status"=w214:bool)
        n94 = property on="Image Message" class="Str"("Visible"=w214) -> ()  [unwired: 2 in, 2 out]
      }
    }
    "Camera Image" <- w201
    n95 = call <vilib>:"WPI_DashboardFormatPerf.vi"("Right Camera Perf"=w194, "Performance"=w195, "String in"=w193) -> ()  [unwired: 9 in]
  }
  n96 = call "Handle Camera Configuration.vi"("CameraNameRef"=w12, "Display Name"=w7, "ClusterRef"=w13) -> ()  [unwired: 9 in]
  n97 = while {
    tunnel: w15 -> [w229]
    tunnel: w14 -> [_]
    tunnel: [w224] -> _
    tunnel: w8 -> [w220]
    tunnel: w7 -> [w217]
    i -> [w224]
    stop <- FALSE stop-if-true
    n98 = local read "NT Connection"() -> (w221:bool)
    n99 = local read "Rec Mode"() -> (w228:enum32{"Stop", "Record", "Playback"})
    n100 = Bundle("Camera Name Right"="Camera Name Right", w217, "Saved DB Images Info"=w220) -> (w219:T19)  [unwired: 1 in]
    n101 = call <vilib>:"WPI_CameraRead MJPG for Dashboard_2.vi"("Camera Settings"="Camera Settings Right", "Rec Mode"=w228, "NT Connection"=w221, "Capture Info"=w219, "Image in"=w229) -> ("perf info"=w215:cluster{"Bandwidth (Mbps)":dbl, "fps":dbl}, "Active"=w223:bool, "Image\\ out"=w226:T6)  [unwired: 4 in]
    n102 = case shown="False" w223 {
      tunnel: w226 -> [w231 w234]
      tunnel: [w231 w234] -> w222
      tunnel: [_ w233] -> w216
      tunnel: w215 -> [_ w233]
      frame False {
        n103 = Wait Until Next ms Multiple(millisecond multiple=u32 500) -> ()  [unwired: 1 out]
        n104 = property on="Camera Image Right" class="ImageControl"("ROI"=T17 {"Global Rectangle"=[], "Contours"=[]}) -> ()  [unwired: 2 in, 2 out]
      }
      frame True {
      }
    }
    "Camera Image Right" <- w222
    "Right Camera Perf" <- w216
  }
  n105 = register-events(refnum<vi> refnum) -> (reference out=w53:refnum<event-registration>, error out=w52:errorcluster)  [unwired: 2 in]
  n106 = call "Initialize Camera and CheckList.vi"("ListBox in"=w39) -> ()  [unwired: 11 in]
  n107 = call "Adjust Dashboard Window_NO_RESIZE.vi"("Sizing Refnums"=w40, "Size Constraints"=w42, "VI"=w49, "WIn Mode"=w27) -> ()  [unwired: 8 in]
  n108 = call <vilib>:"NT Bind Controls to SmartDashboard.vi"("Bound Control Refs"=w47) -> ()  [unwired: 11 in]
  n109 = vi-ref "Playback Controls.vi"() -> (w54:refnum<vi>)
  n110 = property class="VI"() -> ("Panel"=w56:refnum<vi>)  [unwired: 2 in, 2 out]
  n111 = call "FieldDisplaySmall.vi"() -> ()  [unwired: 1 in]
  n112 = property class="Pnl"(reference=w56) -> ("Panes[]"=w57:refnum<vi>[])  [unwired: 1 in, 2 out]
  n113 = Index Array(array=w57) -> (element=w55:refnum<vi>)  [unwired: 1 in]
  n114 = control-ref of="Test Tree"() -> (w58:refnum<vi>)
  n115 = while {
    tunnel: [w240] -> _
    tunnel: w58 -> [w239]
    tunnel: w54 -> [w238]
    tunnel: w53 -> [w237]
    tunnel: w52 -> [_]
    tunnel: w49 -> [w236]
    tunnel: w5 -> [w235]
    i -> [w240]
    stop <- FALSE stop-if-true
    n116 = event shown="[0] Timeout" {
      selector: w237 -> [_ _ _ _ _ _ _ _ _ _ _ _ _ _ _ _ _]
      dyn-events: [_ _ _ _ _ _ _ _ _ _ _ _ _ w447 _ _ _] -> _
      timeout: u32 60 ("milliseconds to wait") -> [_ _ _ _ _ _ _ _ _ _ _ _ _ _ _ _ _]
      tunnel: w239 -> [w250 _ _ _ _ _ _ _ _ _ _ _ _ _ _ _ _]
      tunnel: "Test Tree" -> [_ _ _ _ _ _ _ _ w420 w427 w428 w431 w438 _ _ _ _]
      tunnel: w238 -> [_ _ _ _ _ _ _ _ _ _ _ _ _ w449 _ w464 _]
      tunnel: w236 -> [_ _ _ _ _ _ _ _ _ _ _ _ _ w445 _ _ _]
      tunnel: w235 -> [w245 _ _ _ _ _ _ _ _ _ _ _ _ _ _ _ _]
      event Timeout {
        n117 = event-data() -> ()  [unwired: 1 in, 1 out]
        n118 = local read "Mode"() -> (w248:T5)
        n119 = case shown="\"Variables\"" "Dashboard Tab" {
          tunnel: w250 -> [_ _ w267 _]
          tunnel: "/TestMode/Automatic/" ("Name Pattern") -> [_ _ w266 _]
          tunnel: T20 [{"Operation"=enum."Clear", "Color Box"=14013909}, {"Operation"=enum."Clear", "Color Box"=14013909}, {"Operation"=enum."Clear", "Color Box"=14013909}, {"Operation"=enum."Clear", "Color Box"=14013909}, {"Operation"=enum."Update", "Color Box"=14013909}, {"Operation"=enum."Update", "Color Box"=16777215}, {"Operation"=enum."Clear", "Color Box"=14013909}, {"Operation"=enum."Clear", "Color Box"=14013909}, {"Operation"=enum."Clear", "Color Box"=14013909}] -> [_ _ w259 _]
          tunnel: w248 -> [_ _ w258 _]
          tunnel: u32[] [15790320, 15790320, 15790320, 15790320, 16777215, 16777215, 15790320, 15790320, 15790320] -> [_ _ _ _]
          tunnel: w245 -> [_ w252 _ _]
          frame "Custom", Default {
          }
          frame "Basic" {
            n120 = disable-structure shown="Disabled" {
              disable-tunnel: w252 -> [w253 _]
              frame Disabled {
                n121 = call <vilib>:"WPI_DashboardUpdateNames.vi"("Controls on Tab"=w253) -> ()  [unwired: 11 in]
              }
              frame Enabled {
              }
            }
          }
          frame "Test" {
            w265 = -2 ("Active Item:Row Number")
            n122 = Index Array(array=w259, index=w258) -> (element=w260:T23)
            n123 = Unbundle(w260) -> ("Operation"=w261:enum16{"Update", "Clear"}, "Color Box"=w262:u32)
            n124 = call <vilib>:"NT Read String.vi"("name"="TestMode/TestName" ("Name")) -> ("value"=w256:string)  [unwired: 8 in, 2 out]
            n125 = call <vilib>:"NT Read and Format Entries as Tree.vi"("Operation"=w261, "Name Pattern"=w266, "Tree Refnum"=w267) -> ()  [unwired: 7 in, 2 out]
            n126 = case shown="\"\"" w256 {
              tunnel: "TestMode/TestProgress" ("Name") -> [w269 _]
              tunnel: "TestMode/TestProgressText" ("Name") -> [w268 _]
              frame Default {
                n127 = call <vilib>:"NT Read Number.vi"("name"=w269) -> ("value"=w270:dbl)  [unwired: 8 in, 2 out]
                n128 = call <vilib>:"NT Read String.vi"("name"=w268) -> ("value"=w271:string)  [unwired: 8 in, 2 out]
                n129 = Bundle("value"=w270, "value"=w271) -> (→"Progress":cluster{"value":dbl, "value":string})  [unwired: 1 in]
              }
              frame "" {
                n130 = property on="Progress" class="Clust (strict)"("Visible"=FALSE) -> ()  [unwired: 2 in, 2 out]
                n131 = local write "Test Name"(u16 0) -> ()
              }
            }
            n132 = property on="Test Tree" class="Tree (strict)"("Active Item Row Number"=w265, "ActiveColNum"=w265, "CellBG"=w262, "Active Item Row Number"=-1 ("Active Item:Row Number"), "CellBG"=u32 5789784 ("Color Box")) -> ()  [unwired: 2 in, 2 out]
          }
          frame "Variables" {
            w276 = string[] ["CameraPublisher", "Usage", "DB", "schema", "cameraPublisher", "photonvision"]  # Items to initially close
            # "#NOTE JAS for now..."
            n133 = control-ref of="Tree"() -> (w280:refnum<vi>)
            n134 = First Call?() -> (First Call?: T/F=w279:bool)
            n135 = Select(t=w276, s=w279, f=string[] []) -> (s? t:f=w278:string[])
            n136 = call <vilib>:"NT Read and Format Entries as Tree.vi"("Tags to  Close"=w278, "Name Pattern"="/SmartDashboard/", "Tree Refnum"=w280) -> ()  [unwired: 7 in, 2 out]
          }
        }
        n137 = call <vilib>:"NT Connection Info.vi"() -> ("Connected"=→"NT Connection":bool)  [unwired: 11 in]
      }
      event "Test Tree": Value Change {
        # "Show appropriate\ncontrols"
        n138 = event-data() -> ("CtlRef"=w284:refnum<vi>, "NewVal"=w282:string)  [unwired: 1 in]
        n139 = call <vilib>:"WPI_UtilitiesGetTreeIOName.vi"("NewVal"=w282, "TreeControl in"=w284) -> ("I/O Name"=w285:string)  [unwired: 9 in]
        n140 = case shown="\"Camera\"" w285 {
          selector: w285 -> [_ w292 _ w314 w323 _]
          tunnel: w282 -> [_ _ w311 w313 _ w330]
          tunnel: cluster{string[]}[] [{["640x480", "320x240", "160x120"]}, {["Auto", "Fixed indoor", "Fixed outdoor 1", "Fixed outdoor 2", "Fixed fluorescent 1", "Fixed fluorescent 2", "Hold current"]}, {["Auto", "Flicker-free 50 Hz", "Flicker-free 60 Hz", "Hold current"]}, {["None", "Prioritize frame rate", "Prioritize image quality"]}, {["Monochrome", "Color"]}] -> [_ _ _ _ _ w329]
          frame Default {
            w287 = FALSE ("Visible")
            w286 = FALSE ("Visible")
            n141 = property on="Motor" class="Clust (strict)"("Visible"=w286) -> ()  [unwired: 2 in, 2 out]
            n142 = property on="Test Ring" class="Ring (strict)"("Visible"=w286) -> ()  [unwired: 2 in, 2 out]
            n143 = property on="Rev/Fwd" class="Clust (strict)"("Visible"=w287) -> ()  [unwired: 2 in, 2 out]
            n144 = property on="On/Off" class="Bool (strict)"("Visible"=w287) -> ()  [unwired: 2 in, 2 out]
            n145 = property on="Test Slider" class="Slide (strict)"("Visible"=w287) -> ()  [unwired: 2 in, 2 out]
          }
          frame "Analog Out", "Motor", "PWM" {
            w293 = FALSE ("Visible")
            n146 = case shown="\"Analog Out\"" w292 {
              tunnel: [1.0 ("Value") -1.0 ("Value") 0.0 ("Value")] -> w291
              tunnel: [255.0 ("Value") 1.0 ("Value") 5.0 ("Value")] -> w290
              tunnel: [128.0 ("Value") 0.0 ("Value") 0.0 ("Value")] -> w289
              tunnel: [64.0 ("Value") 0.5 ("Value") 1.0 ("Value")] -> w288
              frame "PWM" {
              }
              frame "Motor", Default {
              }
              frame "Analog Out" {
              }
            }
            n147 = property on="Motor" class="Clust (strict)"("Visible"=TRUE) -> ()  [unwired: 2 in, 2 out]
            n148 = property on="Value" class="Slide (strict)"("Value"=w289, "Scale.Minimum"=w291, "Scale.Maximum"=w290, "Scale.Increment"=w288) -> ()  [unwired: 2 in, 2 out]
            n149 = property on="On/Off" class="Bool (strict)"("Visible"=w293) -> ()  [unwired: 2 in, 2 out]
            n150 = property on="Test Slider" class="Slide (strict)"("Visible"=w293) -> ()  [unwired: 2 in, 2 out]
            n151 = property on="Test Ring" class="Ring (strict)"("Visible"=w293) -> ()  [unwired: 2 in, 2 out]
            n152 = property on="Rev/Fwd" class="Clust (strict)"("Visible"=w293) -> ()  [unwired: 2 in, 2 out]
          }
          frame "Servo" {
            w309 = FALSE ("Visible")
            n153 = call <vilib>:"NT Read Number.vi"("name"=w311) -> ("value"=w310:dbl)  [unwired: 8 in, 2 out]
            n154 = property on="Test Slider" class="Slide (strict)"("Visible"=TRUE, "Scale.Maximum"=170.0 ("Scale.Range:Maximum")) -> ()  [unwired: 2 in, 2 out]
            n155 = local write "Test Slider"(w310) -> ()
            n156 = property on="Motor" class="Clust (strict)"("Visible"=w309) -> ()  [unwired: 2 in, 2 out]
            n157 = property on="Rev/Fwd" class="Clust (strict)"("Visible"=w309) -> ()  [unwired: 2 in, 2 out]
            n158 = property on="On/Off" class="Bool (strict)"("Visible"=w309) -> ()  [unwired: 2 in, 2 out]
            n159 = property on="Test Ring" class="Ring (strict)"("Visible"=w309) -> ()  [unwired: 2 in, 2 out]
          }
          frame "Relay", "Solenoid" {
            w312 = FALSE ("Visible")
            n160 = property on="Motor" class="Clust (strict)"("Visible"=w312) -> ()  [unwired: 2 in, 2 out]
            n161 = property on="Test Slider" class="Slide (strict)"("Visible"=w312) -> ()  [unwired: 2 in, 2 out]
            n162 = Search and Replace String(input string=w313, search string="/Value  **", replace string="/Direction") -> (result string=w319:string)  [unwired: 5 in, 3 out]
            n163 = property on="Test Ring" class="Ring (strict)"("Visible"=w312) -> ()  [unwired: 2 in, 2 out]
            n164 = call <vilib>:"NT Read String.vi"("name"=w319) -> ("value"=w317:string)  [unwired: 8 in, 2 out]
            n165 = Equal?(x="Both directions", y=w317) -> (x = y?=w315:bool)
            n166 = Not(x=w315) -> (.not. x?=w316:bool)
            n167 = property on="Rev/Fwd" class="Clust (strict)"("Visible"=w315) -> ()  [unwired: 2 in, 2 out]
            n168 = property on="On/Off" class="Bool (strict)"("Visible"=w316, "Caption.Text"=w314) -> ()  [unwired: 2 in, 2 out]
          }
          frame "Compressor", "Digital Out" {
            w322 = FALSE ("Visible")
            # "Get direction and finish"
            n169 = property on="Motor" class="Clust (strict)"("Visible"=w322) -> ()  [unwired: 2 in, 2 out]
            n170 = property on="Test Slider" class="Slide (strict)"("Visible"=w322) -> ()  [unwired: 2 in, 2 out]
            n171 = property on="Test Ring" class="Ring (strict)"("Visible"=w322) -> ()  [unwired: 2 in, 2 out]
            n172 = property on="On/Off" class="Bool (strict)"("Visible"=TRUE, "Caption.Text"=w323) -> ()  [unwired: 2 in, 2 out]
            n173 = property on="Rev/Fwd" class="Clust (strict)"("Visible"=FALSE) -> ()  [unwired: 2 in, 2 out]
          }
          frame "Camera" {
            n174 = call <vilib>:"NT_Get Last Path Segment.vi"("String in"=w330) -> ("String out"=w331:string)  [unwired: 10 in]
            n175 = property on="On/Off" class="Bool (strict)"("Visible"=FALSE) -> ()  [unwired: 2 in, 2 out]
            n176 = property on="Motor" class="Clust (strict)"("Visible"=FALSE) -> ()  [unwired: 2 in, 2 out]
            n177 = property on="Rev/Fwd" class="Clust (strict)"("Visible"=FALSE) -> ()  [unwired: 2 in, 2 out]
            n178 = case shown="\"White Balance  **\"" w331 {
              tunnel: w330 -> [w337 w346 w355 w364 w373 _ w379]
              tunnel: w329 -> [w335 w343 w352 w361 w370 _ _]
              frame "Size  **" {
                n179 = Index Array(array=w335) -> (element=w334:cluster{string[]})  [unwired: 1 in]
                n180 = call <vilib>:"NT Read String.vi"("name"=w337) -> ("value"=w336:string)  [unwired: 8 in, 2 out]
                n181 = Unbundle(w334) -> (w332:string[])
                n182 = Match First String(2:w332, 3:w336) -> (0:w333:i32)  [unwired: 1 out]
                n183 = property on="Test Ring" class="Ring (strict)"("Value"=w333, "Strings []"=w332) -> ()  [unwired: 2 in, 2 out]
                n184 = property on="Test Ring" class="Ring (strict)"("Visible"=TRUE) -> ()  [unwired: 2 in, 2 out]
                n185 = property on="Test Slider" class="Slide (strict)"("Visible"=FALSE) -> ()  [unwired: 2 in, 2 out]
              }
              frame "White Balance  **" {
                n186 = Index Array(array=w343, index=1) -> (element=w344:cluster{string[]})
                n187 = call <vilib>:"NT Read String.vi"("name"=w346) -> ("value"=w345:string)  [unwired: 8 in, 2 out]
                n188 = Unbundle(w344) -> (w341:string[])
                n189 = Match First String(2:w341, 3:w345) -> (0:w340:i32)  [unwired: 1 out]
                n190 = property on="Test Ring" class="Ring (strict)"("Value"=w340, "Strings []"=w341) -> ()  [unwired: 2 in, 2 out]
                n191 = property on="Test Ring" class="Ring (strict)"("Visible"=TRUE) -> ()  [unwired: 2 in, 2 out]
                n192 = property on="Test Slider" class="Slide (strict)"("Visible"=FALSE) -> ()  [unwired: 2 in, 2 out]
              }
              frame "Exposure  **" {
                n193 = Index Array(array=w352, index=2) -> (element=w353:cluster{string[]})
                n194 = call <vilib>:"NT Read String.vi"("name"=w355) -> ("value"=w354:string)  [unwired: 8 in, 2 out]
                n195 = Unbundle(w353) -> (w349:string[])
                n196 = Match First String(2:w349, 3:w354) -> (0:w350:i32)  [unwired: 1 out]
                n197 = property on="Test Ring" class="Ring (strict)"("Value"=w350, "Strings []"=w349) -> ()  [unwired: 2 in, 2 out]
                n198 = property on="Test Ring" class="Ring (strict)"("Visible"=TRUE) -> ()  [unwired: 2 in, 2 out]
                n199 = property on="Test Slider" class="Slide (strict)"("Visible"=FALSE) -> ()  [unwired: 2 in, 2 out]
              }
              frame "Exposure Priority  **" {
                n200 = Index Array(array=w361, index=3) -> (element=w362:cluster{string[]})
                n201 = call <vilib>:"NT Read String.vi"("name"=w364) -> ("value"=w363:string)  [unwired: 8 in, 2 out]
                n202 = Unbundle(w362) -> (w358:string[])
                n203 = Match First String(2:w358, 3:w363) -> (0:w359:i32)  [unwired: 1 out]
                n204 = property on="Test Ring" class="Ring (strict)"("Value"=w359, "Strings []"=w358) -> ()  [unwired: 2 in, 2 out]
                n205 = property on="Test Ring" class="Ring (strict)"("Visible"=TRUE) -> ()  [unwired: 2 in, 2 out]
                n206 = property on="Test Slider" class="Slide (strict)"("Visible"=FALSE) -> ()  [unwired: 2 in, 2 out]
              }
              frame "Color Enable  **" {
                n207 = Index Array(array=w370, index=4) -> (element=w371:cluster{string[]})
                n208 = call <vilib>:"NT Read String.vi"("name"=w373) -> ("value"=w372:string)  [unwired: 8 in, 2 out]
                n209 = Unbundle(w371) -> (w367:string[])
                n210 = Match First String(2:w367, 3:w372) -> (0:w368:i32)  [unwired: 1 out]
                n211 = property on="Test Ring" class="Ring (strict)"("Value"=w368, "Strings []"=w367) -> ()  [unwired: 2 in, 2 out]
                n212 = property on="Test Ring" class="Ring (strict)"("Visible"=TRUE) -> ()  [unwired: 2 in, 2 out]
                n213 = property on="Test Slider" class="Slide (strict)"("Visible"=FALSE) -> ()  [unwired: 2 in, 2 out]
              }
              frame Default {
                n214 = property on="Test Ring" class="Ring (strict)"("Visible"=FALSE) -> ()  [unwired: 2 in, 2 out]
                n215 = property on="Test Slider" class="Slide (strict)"("Visible"=FALSE) -> ()  [unwired: 2 in, 2 out]
              }
              frame "Brightness  **", "Color Level  **", "Compression  **", "FPS  **", "Sharpness  **" {
                n216 = call <vilib>:"NT Read Number.vi"("name"=w379) -> ("value"=w378:dbl)  [unwired: 8 in, 2 out]
                n217 = local write "Test Slider"(w378) -> ()
                n218 = property on="Test Ring" class="Ring (strict)"("Visible"=FALSE) -> ()  [unwired: 2 in, 2 out]
                n219 = property on="Test Slider" class="Slide (strict)"("Visible"=TRUE, "Scale.Maximum"=100.0 ("Scale.Range:Maximum")) -> ()  [unwired: 2 in, 2 out]
              }
            }
          }
        }
        n220 = property on="Progress" class="Clust (strict)"("Visible"=FALSE) -> ()  [unwired: 2 in, 2 out]
      }
      event "Test Name": Mouse Enter {
        # "Populate the ring with the list of tests"
        n221 = event-data() -> ()  [unwired: 1 in, 1 out]
        n222 = call <vilib>:"NT Read String Array.vi"("name"="TestMode/TestList" ("Name")) -> ("value"=w386:string[])  [unwired: 8 in, 2 out]
        n223 = Build Array (concatenate)("Select the test to run...", w386) -> (w385:string[])
        n224 = property on="Test Name" class="Ring (strict)"("Strings []"=w385) -> ()  [unwired: 2 in, 2 out]
      }
      event "Test Name": Value Change {
        w387 = FALSE ("Visible")
        # "Tell the robot the test name to run"
        n225 = event-data() -> ("NewVal"=w391:u16)  [unwired: 1 in]
        n226 = property on="Test Name" class="Ring (strict)"() -> ("Strings []"=w392:string[])  [unwired: 2 in, 2 out]
        n227 = local write "Progress"(T8 {"Test Progress"=0, "Test Progress Text"=""} ("Progress")) -> ()
        n228 = Index Array(array=w392, index=w391) -> (element=w390:string)
        n229 = call <vilib>:"NT Write String.vi"("value"=w390, "name"="TestMode/TestName" ("Name")) -> ()  [unwired: 9 in, 1 out]
        n230 = property on="Progress" class="Clust (strict)"("Visible"=TRUE) -> ()  [unwired: 2 in, 2 out]
        n231 = property on="Motor" class="Clust (strict)"("Visible"=w387) -> ()  [unwired: 2 in, 2 out]
        n232 = property on="Test Slider" class="Slide (strict)"("Visible"=w387) -> ()  [unwired: 2 in, 2 out]
        n233 = property on="On/Off" class="Bool (strict)"("Visible"=w387) -> ()  [unwired: 2 in, 2 out]
        n234 = property on="Rev/Fwd" class="Clust (strict)"("Visible"=w387) -> ()  [unwired: 2 in, 2 out]
        n235 = property on="Test Ring" class="Ring (strict)"("Visible"=w387) -> ()  [unwired: 2 in, 2 out]
      }
      event "Select Auto": Mouse Enter {
        # "Populate the combo box with the list of autonomous options"
        n236 = event-data() -> ()  [unwired: 1 in, 1 out]
        n237 = call <vilib>:"NT Read String Array.vi"("name"="Auto List" ("Name")) -> ("value"=w394:string[])  [unwired: 8 in, 2 out]
        n238 = property on="Select Auto" class="CmbBox"("Strings[]"=w394) -> ()  [unwired: 2 in, 2 out]
      }
      event "Select Auto": Value Change {
        # "User modified the Auto Selection. Write to NT variable so robot knows."
        n239 = event-data() -> ("NewVal"=w396:string)  [unwired: 1 in]
        n240 = call <vilib>:"NT Write String.vi"("value"=w396, "name"="Auto Selector" ("Name")) -> ()  [unwired: 9 in, 1 out]
      }
      event "CheckList": Double Click {
        # "Shift clears all"
        # "Update symbols on the listbox"
        n241 = event-data() -> ("PlatMods.Shift"=w398:bool, "Row"=w400:i32)  [unwired: 1 in]
        n242 = case shown="True" w398 {
          tunnel: w400 -> [w404 _]
          tunnel: 1 -> [w403 _]
          frame False {
            n243 = property on="CheckList" class="LstBox (strict)"() -> ("Item Symbols"=w402:i32[])  [unwired: 2 in, 2 out]
            n244 = Replace Array Subset(array=w402, new element=w403, index=w404) -> (w401:i32[])
            n245 = property on="CheckList" class="LstBox (strict)"("Item Symbols"=w401) -> ()  [unwired: 2 in, 2 out]
          }
          frame True {
            w405 = 0 ("Top Row")
            n246 = property on="CheckList" class="LstBox (strict)"() -> ("Number of Rows"=w407:u32)  [unwired: 2 in, 2 out]
            n247 = Initialize Array(0, w407) -> (w406:i32[])
            n248 = property on="CheckList" class="LstBox (strict)"("Top Row"=w405, "Value"=w405, "Item Symbols"=w406) -> ()  [unwired: 2 in, 2 out]
          }
        }
      }
      event "CheckList": Key Down {
        # "Update symbols on the listbox\nLeft and right keys check and uncheck"
        n249 = event-data() -> ("VKey"=w410:T21)  [unwired: 1 in]
        n250 = case shown="\"Left\", \"Right\"" w410 {
          selector: w410 -> [w415 _]
          tunnel: eventvkey."Left" ("VKey") -> [w413 _]
          frame "Left", "Right" {
            n251 = Equal?(x=w413, y=w415) -> (x = y?=w414:bool)
            n252 = Select(t=0, s=w414, f=1) -> (s? t:f=w416:i32)
            n253 = property on="CheckList" class="LstBox (strict)"() -> ("Item Symbols"=w419:i32[])  [unwired: 2 in, 2 out]
            n254 = Replace Array Subset(array=w419, new element=w416, index="CheckList") -> (w418:i32[])
            n255 = property on="CheckList" class="LstBox (strict)"("Item Symbols"=w418) -> ()  [unwired: 2 in, 2 out]
          }
          frame Default {
          }
        }
      }
      event "Motor.Enable": Value Change {
        # "When the test mode otor enable helper is set, update that\ntree row item's value"
        n256 = event-data() -> ("NewVal"=w424:bool)  [unwired: 1 in]
        n257 = Unbundle("Motor") -> ("Value"=w423:dbl)  [unwired: 1 out]
        n258 = Select(t=w423, s=w424, f=0.0) -> (s? t:f=w421:dbl)
        n259 = call <vilib>:"NT Write Number.vi"("value"=w421, "name"=w420) -> ()  [unwired: 9 in, 1 out]
      }
      event "Test Slider": Value Change {
        # "When the test mode slider helper is set, update that\ntree row item's value"
        n260 = event-data() -> ("NewVal"=w426:dbl)  [unwired: 1 in]
        n261 = call <vilib>:"NT Write Number.vi"("value"=w426, "name"=w427) -> ()  [unwired: 9 in, 1 out]
      }
      event "On/Off": Value Change {
        # "When the test mode on/off helper value is set, update that\ntree row item's value"
        n262 = event-data() -> ("NewVal"=w430:bool)  [unwired: 1 in]
        n263 = Boolean To (0,1)(Boolean=w430) -> (0, 1=w429:i16)
        n264 = call <vilib>:"NT Write Number.vi"("value"=w429, "name"=w428) -> ()  [unwired: 9 in, 1 out]
      }
      event "Rev/Fwd": Value Change {
        # "When the test mode helper value for relays is set, update that\ntree row item's value"
        n265 = event-data() -> ("NewVal.Forward"=w437:bool, "NewVal.Reverse"=w436:bool)  [unwired: 1 in]
        n266 = Boolean To (0,1)(Boolean=w437) -> (0, 1=w433:i16)
        n267 = Boolean To (0,1)(Boolean=w436) -> (0, 1=w435:i16)
        n268 = Negate(x=w435) -> (-x=w434:i16)
        n269 = Add(x=w433, y=w434) -> (x+y=w432:i16)
        n270 = call <vilib>:"NT Write Number.vi"("value"=w432, "name"=w431) -> ()  [unwired: 9 in, 1 out]
      }
      event "Test Ring": Value Change {
        # "When a test mode helper value is selected from the ring,\nset the tree item's variable to the string value"
        n271 = event-data() -> ("NewVal"=w440:u16)  [unwired: 1 in]
        n272 = property on="Test Ring" class="Ring (strict)"() -> ("Strings []"=w441:string[])  [unwired: 2 in, 2 out]
        n273 = Index Array(array=w441, index=w440) -> (element=w439:string)
        n274 = call <vilib>:"NT Write String.vi"("value"=w439, "name"=w438) -> ()  [unwired: 9 in, 1 out]
      }
      event "Rec Mode": Value Change {
        # "Update globals for recording mode and path to read log from.\nClear when logging and let NetworkTables set path for vision to\nuse."
        n275 = event-data() -> ("NewVal"=w450:enum32{"Stop", "Record", "Playback"})  [unwired: 1 in]
        n276 = global write "WPI_DashboardLogging Global.vi" "Logging Filename"(path "") -> ()
        n277 = global write "WPI_DashboardLogging Global.vi" "Recording"(w450) -> ()
        n278 = case shown="\"Playback\"" w450 {
          tunnel: w449 -> [_ w452 w460]
          tunnel: [_ _ w459] -> w447
          tunnel: [_ _ w458] -> _
          tunnel: w445 -> [_ _ w456]
          tunnel: cluster{i32, i32} {-250, 170} -> [_ _ w455]
          tunnel: [_ _ T22 {"Image Size"=TRUE, "Image Type"=TRUE, "Pixel Value"=TRUE, "ROI Information"=TRUE, "Zoom Factor"=FALSE} ("Image Information Shown:All Elements")] -> w442
          tunnel: [_ _ TRUE ("Zoom Factor")] -> w443
          frame Default {
          }
          frame "Stop", "Record" {
            # "Place Window too"
            n279 = invoke class="VI" method="FP.Close"(reference=w452) -> (reference out=w451:refnum<vi>)  [unwired: 2 in, 2 out]
            n280 = invoke class="VI" method="Abort VI"(reference=w451) -> ()  [unwired: 2 in, 3 out]
          }
          frame "Playback" {
            n281 = call "Open Playback Panel.vi"("Offset"=w455, "DB VI Ref"=w456, "Playback in"=w460) -> ("Playback out"=w457:refnum<vi>)  [unwired: 8 in]
            n282 = register-events(w457) -> (reference out=w459:refnum<event-registration>, error out=w458:errorcluster)  [unwired: 2 in]
          }
        }
        n283 = property on="Camera Image Right" class="ImageControl"("Image Information Shown"=w442, "Image Information Visible"=w443) -> ()  [unwired: 2 in, 2 out]
        n284 = property on="Camera Image" class="ImageControl"("Image Information Shown"=w442, "Image Information Visible"=w443) -> ()  [unwired: 2 in, 2 out]
        n285 = call <vilib>:"WPI_DashboardNT Log FieldName Cache.vi"("Operation"=enum16{"Lookup/Add", "Index", "Clear"}."Clear") -> ()  [unwired: 8 in, 3 out]
      }
      event Panel Close {
        w461 = enum32{"Stop", "Record", "Playback"}."Stop" ("Rec Mode")
        # "Playback window has been closed, abort"
        n286 = event-data() -> ()  [unwired: 1 in, 4 out]
        n287 = local write "Rec Mode"(w461) -> ()
        n288 = global write "WPI_DashboardLogging Global.vi" "Recording"(w461) -> ()
      }
      event Panel Close {
        # "Abort playback window and ourself"
        n289 = event-data() -> ()  [unwired: 1 in, 4 out]
        n290 = invoke class="VI" method="FP.Close"(reference=w464) -> (reference out=w463:refnum<vi>)  [unwired: 2 in, 2 out]
        n291 = invoke class="VI" method="Abort VI"(reference=w463) -> (error out=w462:errorcluster)  [unwired: 2 in, 2 out]
        n292 = invoke class="VI" method="Abort VI"(error in=w462) -> ()  [unwired: 2 in, 3 out]
      }
      event "Tree": Double Click {
        n293 = event-data() -> ("PlatMods"=w470:T24, "Tag"=w467:string)  [unwired: 1 in]
        n294 = Unbundle(w470) -> ("Shift"=w469:bool)  [unwired: 4 out]
        n295 = String Subset(string=w467, length (rest)=1 ("length (rest)")) -> (substring=w466:string)  [unwired: 1 in]
        n296 = Not(x=w469) -> (.not. x?=w468:bool)
        n297 = case shown="\"/\"" w466 {
          tunnel: w467 -> [_ w472]
          tunnel: w468 -> [_ w471]
          frame Default {
          }
          frame "/" {
            n298 = call <vilib>:"NT Update Persistence.vi"("Persistence"=w471, "Name"=w472) -> ()  [unwired: 9 in, 1 out]
          }
        }
      }
    }
  }
  n299 = while {
    tunnel: w55 -> [w474]
    i -> [w477]
    stop <- FALSE stop-if-true
    n300 = Wait (ms)(milliseconds to wait=u32 100) -> ()  [unwired: 1 out]
    n301 = case shown="\"Playback\"" "Rec Mode" {
      tunnel: w477 -> [_ _ w492]
      tunnel: [u32 2829099 ("Base Color") u32 11141120 ("Target Color") w481] -> w473
      frame "Stop", Default {
        # "Reset the color, extra updates don't cost much"
      }
      frame "Record" {
      }
      frame "Playback" {
        # "Playback"
        n302 = Quotient & Remainder(x=w492, y=u32 50 ("milliseconds to wait")) -> (x-y*floor(x/y)=w488:u32)  [unwired: 1 out]
        n303 = Divide(x=w488, y=u32 50 ("milliseconds to wait")) -> (x/y=w485:dbl)
        n304 = Multiply(x=6.283185307179586, y=w485) -> (x*y=w490:dbl)
        n305 = Sine(x=w490) -> (sin(x)=w489:dbl)
        n306 = Absolute Value(x=w489) -> (abs(x)=w482:dbl)
        n307 = call "Interpolate RGB Color.vi"("Proportion"=w482, "Target Color"=u32 30976, "Base Color"=u32 2829099) -> ("Result Color"=w481:u32)  [unwired: 8 in]
      }
    }
    n308 = property class="Pane"(reference=w474, "PaneColor"=w473) -> ()  [unwired: 1 in, 2 out]
  }
  n309 = call "DriveModuleTrend.vi"("Module"=0) -> ()  [unwired: 11 in]
  n310 = call "DriveModuleTrend.vi"("Module"=1) -> ()  [unwired: 11 in]
  n311 = call "DriveModuleTrend.vi"("Module"=2) -> ()  [unwired: 11 in]
  n312 = local write "Dashboard Tab"(T2."Drive" ("Dashboard Tab")) -> ()
  n313 = call "DriveModuleTrend.vi"("Module"=3) -> ()  [unwired: 11 in]
  n314 = call "TrajectoryTrend.vi"() -> ()  [unwired: 12 in]
  n315 = property on="On/Off" class="Bool (strict)"("Visible"=w28) -> ()  [unwired: 2 in, 2 out]
  n316 = property on="Motor" class="Clust (strict)"("Visible"=w28) -> ()  [unwired: 2 in, 2 out]
  n317 = property on="Progress" class="Clust (strict)"("Visible"=w28) -> ()  [unwired: 2 in, 2 out]
  n318 = property on="Test Ring" class="Ring (strict)"("Visible"=w28) -> ()  [unwired: 2 in, 2 out]
  n319 = property on="Rev/Fwd" class="Clust (strict)"("Visible"=w28) -> ()  [unwired: 2 in, 2 out]
  n320 = while {
    tunnel: u16 1741 ("timeout ms (25000)") -> [w494]
    stop <- FALSE stop-if-true
    n321 = TCP Create Listener(10:w494) -> (0:w493:errorcluster, 3:w495:refnum<k5>)  [unwired: 4 in, 1 out]
    n322 = case shown="No Error" w493 {
      selector: w493 -> [w497 _]
      tunnel: w495 -> [w498 _]
      frame No Error {
        n323 = while {
          tunnel: w498 -> [w501]
          tunnel: w497 -> [w500]
          stop <- FALSE stop-if-true
          n324 = TCP Wait On Listener(8:w500, 11:w501) -> (0:w502:errorcluster, 4:w503:refnum<k5>)  [unwired: 2 in, 3 out]
          n325 = local write "TCP"(w503) -> ()
          n326 = case shown="Error" w502 {
            frame No Error {
            }
            frame Error {
              n327 = Wait (ms)(milliseconds to wait=u32 1000) -> ()  [unwired: 1 out]
            }
          }
        }
      }
      frame Error {
        n328 = Wait (ms)(milliseconds to wait=u32 1000) -> ()  [unwired: 1 out]
      }
    }
  }
  n329 = global write "WPI_DashboardLogging Global.vi" "Recording"(w50) -> ()
  n330 = local write "Rec Mode"(w50) -> ()
  n331 = call <vilib>:"NT Write String.vi"("value"="Select Auto", "name"="Auto Selector" ("Name")) -> ()  [unwired: 9 in, 1 out]
